vi "Get_Loop_Iteration.vi"(1 "Loop Count":cluster{string, "Position":i32}[](array[cluster]), 2 "Loop Event":cluster{string, string[], dbl[], dbl}) -> (0 "Iteration Descriptor":string)   [LabVIEW 2011]
doc: "This VI returns the a string designed to inform the user of the current iteration number of a given loop, as well as the total number of iterations of that loop."
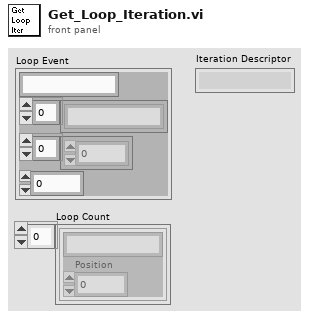
[diagram p1: front panel]
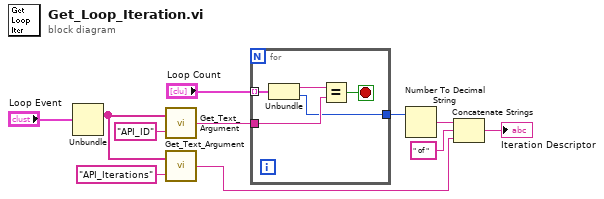
[diagram p0: block diagram]
diagram:
  n1 = Unbundle("Loop Event") -> (w8:string[])  [unwired: 3 out]
  n2 = call "Get_Text_Argument.vi"("Argument"="API_ID", "Argument List"=w8) -> ("Text"=w7:string)
  n3 = call "Get_Text_Argument.vi"("Argument"="API_Iterations", "Argument List"=w8) -> ("Text"=w2:string)
  n4 = for {
    tunnel: w7 -> [w14]
    tunnel: "Loop Count" -> [w16] mode=indexing
    tunnel: [w13] -> w5
    stop <- w12 stop-if-true
    n5 = Unbundle(w16) -> (w15:string, "Position"=w13:i32)
    n6 = Equal?(x=w15, y=w14) -> (x = y?=w12:bool)
  }
  n7 = Number To Decimal String(number=w5) -> (decimal integer string=w4:string)  [unwired: 1 in]
  n8 = Concatenate Strings(w4, " of " ("string"), w2) -> (→"Iteration Descriptor":string)
